vi "C to F.vi"(8 "error in (no error)":errorcluster) -> (0 "error out":errorcluster, 2 "x+y":dbl, 3 "number":dbl)   [LabVIEW 2023]
uses:
  <vilib>/numeric/Random Number (Range) U64.vi
  <vilib>/numeric/sub_Random U32.vi
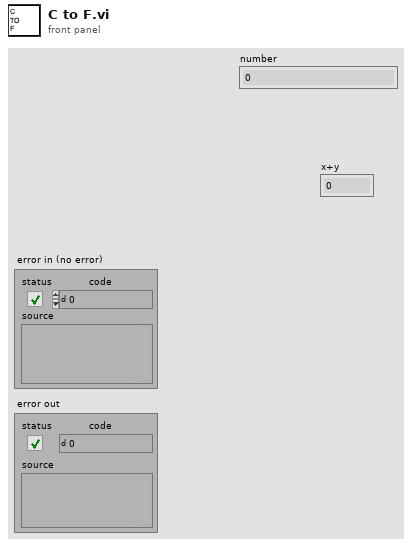
[diagram p1: front panel]
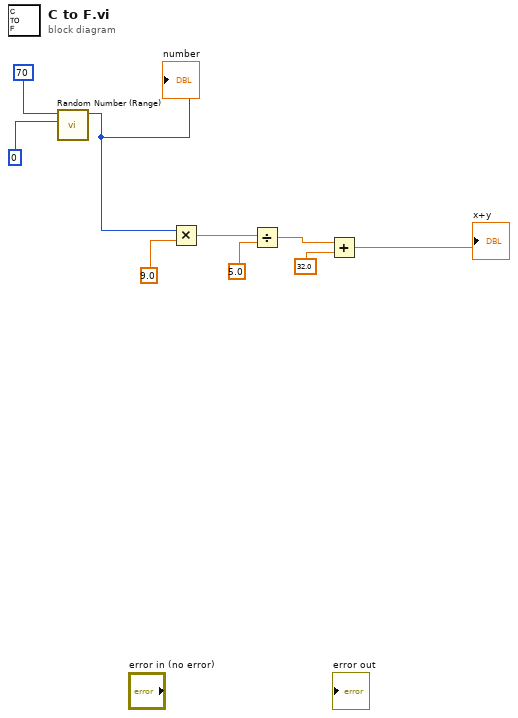
[diagram p0: block diagram]
diagram:
  n1 = call-poly <vilib>:"Random Number (Range).vi"("lower bound (0)"=u64 0, "upper bound (100)"=u64 70) -> ("number"=w1:u64)  [unwired: 9 in]
  "number" <- w1
  n2 = Multiply(x=w1, y=9.0) -> (x*y=w8:dbl)
  n3 = Divide(x=w8, y=5.0) -> (x/y=w6:dbl)
  n4 = Add(x=w6, y=32.0) -> (x+y=→"x+y":dbl)
